vi "HFRR ADV v023 new software.vi"() -> ()   [LabVIEW 2025] (continued)
                  n3402 = property on="WS1.4" class="DigNum (strict)"("Caption.Text"=w4564) -> ()  [unwired: 2 in, 2 out]
                }
                frame 45 {
                  n3403 = property on="Save Results" class="Bool (strict)"("Boolean Text.Text"=w4566) -> ()  [unwired: 2 in, 2 out]
                }
                frame 46 {
                  n3404 = local write "S 47"(w4567) -> ()
                }
                frame 47 {
                  n3405 = local write "S 48"(w4568) -> ()
                }
                frame 48 {
                  n3406 = local write "S 49"(w4569) -> ()
                }
                frame 49 {
                  n3407 = local write "S 50"(w4570) -> ()
                }
                frame 50 {
                  n3408 = local write "S 51"(w4571) -> ()
                }
                frame 51 {
                  n3409 = local write "S 52"(w4572) -> ()
                }
                frame 52 {
                  n3410 = local write "S 53"(w4573) -> ()
                }
                frame 53 {
                  n3411 = local write "S 54"(w4574) -> ()
                }
                frame 54 {
                  n3412 = local write "S 55"(w4575) -> ()
                }
                frame 55 {
                  n3413 = local write "S 56"(w4576) -> ()
                }
                frame 56 {
                  n3414 = local write "S 57"(w4577) -> ()
                }
                frame 57 {
                  n3415 = local write "S 58"(w4578) -> ()
                }
                frame 58 {
                  n3416 = local write "S 59"(w4579) -> ()
                }
                frame 59 {
                  n3417 = local write "S 60"(w4580) -> ()
                }
                frame 60 {
                  n3418 = local write "S 62"(w4581) -> ()
                }
                frame 61 {
                  n3419 = local write "S 63"(w4582) -> ()
                }
                frame 62 {
                  n3420 = local write "S 64"(w4583) -> ()
                }
                frame 63 {
                  n3421 = local write "S 65"(w4584) -> ()
                }
                frame 64 {
                  n3422 = local write "S 66"(w4585) -> ()
                }
                frame 65 {
                  n3423 = local write "S 67"(w4586) -> ()
                }
                frame 66 {
                  n3424 = local write "S 68"(w4587) -> ()
                }
                frame 67 {
                  n3425 = local write "S 69"(w4588) -> ()
                }
                frame 68 {
                  n3426 = local write "S 70"(w4589) -> ()
                }
                frame 69 {
                  n3427 = local write "S 71"(w4590) -> ()
                }
                frame 70 {
                  n3428 = local write "S 72"(w4591) -> ()
                }
                frame 71 {
                  n3429 = local write "S 73"(w4592) -> ()
                }
                frame 72 {
                  n3430 = local write "S 74"(w4593) -> ()
                }
                frame 73 {
                  n3431 = local write "S 75"(w4594) -> ()
                }
                frame 74 {
                  n3432 = local write "S 76"(w4595) -> ()
                }
                frame 75 {
                  n3433 = local write "S 77"(w4596) -> ()
                }
                frame 76 {
                  n3434 = local write "S 78"(w4597) -> ()
                }
                frame 77 {
                  n3435 = local write "S 79"(w4598) -> ()
                }
                frame 79 {
                  n3436 = property on="Sample Temperature ( °C )" class="XYGraph (strict)"("Y Scale.Name Label.Text"=w4599) -> ()  [unwired: 2 in, 2 out]
                }
                frame 80 {
                  n3437 = local write "S 81"(w4600) -> ()
                  n3438 = property on="Humidity ( %RH )" class="XYGraph (strict)"("Y Scale.Name Label.Text"=w4600) -> ()  [unwired: 2 in, 2 out]
                }
                frame 78 {
                  n3439 = property on="Air Temperature  ( °C )" class="XYGraph (strict)"("X Scale.Name Label.Text"=w4601) -> ()  [unwired: 2 in, 2 out]
                  n3440 = property on="Humidity ( %RH )" class="XYGraph (strict)"("X Scale.Name Label.Text"=w4601) -> ()  [unwired: 2 in, 2 out]
                  n3441 = property on="Sample Temperature ( °C )" class="XYGraph (strict)"("X Scale.Name Label.Text"=w4601) -> ()  [unwired: 2 in, 2 out]
                  n3442 = property on="Coefficient Of Friction" class="XYGraph (strict)"("X Scale.Name Label.Text"=w4601) -> ()  [unwired: 2 in, 2 out]
                }
                frame 81 {
                  n3443 = property on="Air Temperature  ( °C )" class="XYGraph (strict)"("Y Scale.Name Label.Text"=w4602) -> ()  [unwired: 2 in, 2 out]
                }
                frame 82 {
                  n3444 = local write "S 84"(w4603) -> ()
                }
                frame 83 {
                  n3445 = local write "S 85"(w4604) -> ()
                }
                frame 84 {
                  n3446 = local write "S 86"(w4605) -> ()
                }
                frame 85 {
                  n3447 = local write "S 87"(w4606) -> ()
                }
                frame 86 {
                  n3448 = local write "S 88"(w4607) -> ()
                }
                frame 87 {
                }
                frame 88 {
                  n3449 = local write "S 90"(w4609) -> ()
                }
                frame 89 {
                  n3450 = local write "S 91"(w4610) -> ()
                }
                frame 90 {
                  n3451 = local write "S 92"(w4611) -> ()
                }
                frame 91 {
                  n3452 = local write "S 93"(w4612) -> ()
                }
                frame 92 {
                  n3453 = local write "S 94"(w4613) -> ()
                }
                frame 93 {
                  n3454 = local write "S 95"(w4614) -> ()
                }
                frame 94 {
                  n3455 = local write "S 96"(w4615) -> ()
                }
                frame 95 {
                  n3456 = local write "S 97"(w4616) -> ()
                }
                frame 96 {
                  n3457 = local write "S 98"(w4617) -> ()
                }
                frame 97 {
                  n3458 = local write "S 99"(w4618) -> ()
                }
                frame 98 {
                  n3459 = local write "S 100"(w4619) -> ()
                }
                frame 99 {
                  n3460 = local write "S 101"(w4620) -> ()
                }
                frame 100 {
                  n3461 = local write "S 102"(w4621) -> ()
                }
                frame 101 {
                  n3462 = local write "S 103"(w4622) -> ()
                }
                frame 102 {
                  n3463 = local write "S 104"(w4623) -> ()
                }
                frame 103 {
                  n3464 = local write "S 105"(w4624) -> ()
                }
                frame 104 {
                  n3465 = local write "S 106"(w4625) -> ()
                }
                frame 105 {
                }
                frame 106 {
                  n3466 = property on="OK Button 17" class="Bool (strict)"("Boolean Text.Text"=w4626) -> ()  [unwired: 2 in, 2 out]
                }
                frame 107 {
                  n3467 = property on="OK Button 16" class="Bool (strict)"("Boolean Text.Text"=w4627) -> ()  [unwired: 2 in, 2 out]
                }
                frame 108 {
                  n3468 = property on="TITTLE" class="Str"("Caption.Text"=w4628) -> ()  [unwired: 2 in, 2 out]
                }
                frame 109 {
                  "String 30" <- w4629
                }
                frame 110 {
                  n3469 = property on="Test Date" class="Str"("Caption.Text"=w4630) -> ()  [unwired: 2 in, 2 out]
                  "String 31" <- w4630
                }
                frame 111 {
                  n3470 = property on="Sample ID" class="Str"("Caption.Text"=w4631) -> ()  [unwired: 2 in, 2 out]
                  "String 32" <- w4631
                }
                frame 112 {
                  n3471 = property on="Tested by" class="Str"("Caption.Text"=w4632) -> ()  [unwired: 2 in, 2 out]
                  "String 33" <- w4632
                }
                frame 113 {
                  n3472 = property on="System Configured Printers 2" class="Arr (strict)"("Caption.Text"=w4633) -> ()  [unwired: 2 in, 2 out]
                }
                frame 114 {
                  n3473 = property on="Selected Printer" class="Str"("Caption.Text"=w4634) -> ()  [unwired: 2 in, 2 out]
                }
                frame 115 {
                  n3474 = property on="Select Printer 3" class="DigNum (strict)"("Caption.Text"=w4635) -> ()  [unwired: 2 in, 2 out]
                }
                frame 116 {
                  n3475 = property on="Print" class="Bool (strict)"("Boolean Text.Text"=w4636) -> ()  [unwired: 2 in, 2 out]
                }
                frame 117 {
                  "String 41" <- w4637
                }
                frame 118 {
                  n3476 = property on="tested by" class="Str"("Caption.Text"=w4638) -> ()  [unwired: 2 in, 2 out]
                }
                frame 119 {
                }
                frame 120 {
                  n3477 = property on="Export" class="Bool (strict)"("Boolean Text.Text"=w4639) -> ()  [unwired: 2 in, 2 out]
                }
                frame 121 {
                  n3478 = property on="TEMP INTERCEPT:" class="DigNum (strict)"("Caption.Text"=w4640) -> ()  [unwired: 2 in, 2 out]
                }
                frame 122 {
                  n3479 = property on="AIR TEMP INTERCEPT:" class="DigNum (strict)"("Caption.Text"=w4641) -> ()  [unwired: 2 in, 2 out]
                }
                frame 123 {
                  n3480 = property on="Select File Type" class="Enum (strict)"("Caption.Text"=w4642) -> ()  [unwired: 2 in, 2 out]
                }
                frame 124 {
                  n3481 = property on="s.NO" class="Str"("Caption.Text"=w4643) -> ()  [unwired: 2 in, 2 out]
                  "String 45" <- w4643
                }
                frame 125 {
                  n3482 = property on="trip1 8" class="Bool (strict)"("Boolean Text.Text"=w4644) -> ()  [unwired: 2 in, 2 out]
                }
                frame 126, Default {
                }
              }
            }
          }
          frame #1 {
            w4652 = TRUE ("Visible")
            n3483 = local read "S 91"() -> (w4669:string)
            n3484 = local read "S 90"() -> (w4668:string)
            n3485 = local read "S 88"() -> (w4667:string)
            n3486 = property on="File Path" class="Path"("Caption.Text"=w4668) -> ()  [unwired: 2 in, 2 out]
            n3487 = property on="SrvM CP" class="Bool (strict)"("Boolean Text.Text"=w4667) -> ()  [unwired: 2 in, 2 out]
            n3488 = local read "S 71"() -> (w4662:string)
            n3489 = local read "S 86"() -> (w4664:string)
            n3490 = local read "S 85"() -> (w4665:string)
            n3491 = local read "S 87"() -> (w4663:string)
            n3492 = local read "S 84"() -> (w4666:string)
            n3493 = local read "S 103"() -> (w4651:string)
            n3494 = local read "S 104"() -> (w4650:string)
            n3495 = property on="ENTER THE NEW PASSWORD" class="Str"("Caption.Text"=w4663) -> ()  [unwired: 2 in, 2 out]
            n3496 = property on="Password" class="Str"("Caption.Text"=w4665) -> ()  [unwired: 2 in, 2 out]
            n3497 = property on="ENTER CURRENT PASSWORD" class="Str"("Caption.Text"=w4664) -> ()  [unwired: 2 in, 2 out]
            n3498 = property on="EDIT" class="Bool (strict)"("Boolean Text.Text"=w4662) -> ()  [unwired: 2 in, 2 out]
            n3499 = property on="SAVE" class="Bool (strict)"("Boolean Text.Text"=w4666) -> ()  [unwired: 2 in, 2 out]
            n3500 = Build Array(w4651, w4650) -> (w4649:string[])
            n3501 = property on="Heater Button" class="Bool (strict)"("Strings [4]"=w4649) -> ()  [unwired: 2 in, 2 out]
            n3502 = property on="CH-HUMIDITY WET" class="DigNum (strict)"("Caption.Size to Text?"=w4652) -> ()  [unwired: 2 in, 2 out]
            n3503 = property on="CH-HUMIDITY DRY" class="DigNum (strict)"("Caption.Size to Text?"=w4652) -> ()  [unwired: 2 in, 2 out]
            n3504 = property on="CH-POWER -" class="DigNum (strict)"("Caption.Size to Text?"=w4652) -> ()  [unwired: 2 in, 2 out]
            n3505 = property on="CH-HEATER" class="DigNum (strict)"("Caption.Size to Text?"=w4652) -> ()  [unwired: 2 in, 2 out]
            n3506 = property on="CH-POWER +" class="DigNum (strict)"("Caption.Size to Text?"=w4652) -> ()  [unwired: 2 in, 2 out]
            n3507 = local read "S 92"() -> (w4661:string)
            n3508 = local read "S 93"() -> (w4660:string)
            n3509 = local read "S 105"() -> (w4647:string)
            n3510 = local read "S 106"() -> (w4646:string)
            n3511 = Build Array(w4661, w4660) -> ()  [unwired: 1 out]
            n3512 = Build Array(w4647, w4646) -> (w4648:string[])
            n3513 = local read "S 95"() -> (w4658:string)
            n3514 = local read "S 94"() -> (w4659:string)
            n3515 = local read "bs"() -> (w4674:string)
            n3516 = local read "as"() -> (w4675:string)
            n3517 = property on="Humidity" class="Bool (strict)"("Strings [4]"=w4648) -> ()  [unwired: 2 in, 2 out]
            n3518 = Concatenate Strings(w4674, "\r", w4675) -> ()  [unwired: 1 out]
            n3519 = property on="STROKE GAIN :" class="DigNum (strict)"("Caption.Text"=w4658) -> ()  [unwired: 2 in, 2 out]
            n3520 = property on="DISPLACEMENT :" class="DigNum (strict)"("Caption.Text"=w4659) -> ()  [unwired: 2 in, 2 out]
            n3521 = property on="Rh After" class="DigNum (strict)"("Caption.Size to Text?"=TRUE ("Caption.Size to Text")) -> ()  [unwired: 2 in, 2 out]
            n3522 = local read "S 48"() -> (w4698:string)
            n3523 = local read "S 50"() -> (w4696:string)
            n3524 = local read "S 51"() -> (w4695:string)
            n3525 = local read "S 49"() -> (w4697:string)
            n3526 = local read "S 52"() -> (w4694:string)
            n3527 = local read "as"() -> (w4679:string)
            n3528 = local read "bs"() -> (w4680:string)
            n3529 = local read "S 56"() -> (w4693:string)
            n3530 = local read "S 57"() -> (w4692:string)
            n3531 = local read "S 58"() -> (w4691:string)
            n3532 = local read "S 59"() -> (w4690:string)
            n3533 = property on="OPEN" class="Bool (strict)"("Boolean Text.Text"=w4694) -> ()  [unwired: 2 in, 2 out]
            n3534 = property on="OPEN 1" class="Bool (strict)"("Boolean Text.Text"=w4698) -> ()  [unwired: 2 in, 2 out]
            n3535 = property on="OPEN 2" class="Bool (strict)"("Boolean Text.Text"=w4697) -> ()  [unwired: 2 in, 2 out]
            n3536 = property on="OPEN 3" class="Bool (strict)"("Boolean Text.Text"=w4696) -> ()  [unwired: 2 in, 2 out]
            n3537 = property on="OPEN 4" class="Bool (strict)"("Boolean Text.Text"=w4695) -> ()  [unwired: 2 in, 2 out]
            n3538 = Concatenate Strings(w4680, "\r", w4679) -> ()  [unwired: 1 out]
            n3539 = local read "S 102"() -> (w4653:string)
            n3540 = property on="КОФ1" class="DigNum (strict)"("Caption.Text"=w4693) -> ()  [unwired: 2 in, 2 out]
            n3541 = local read "S 98"() -> (w4657:string)
            n3542 = local read "S 99"() -> (w4656:string)
            n3543 = local read "S 100"() -> (w4655:string)
            n3544 = local read "S 101"() -> (w4654:string)
            n3545 = property on="КОФ2" class="DigNum (strict)"("Caption.Text"=w4692) -> ()  [unwired: 2 in, 2 out]
            n3546 = property on="КОФ3" class="DigNum (strict)"("Caption.Text"=w4691) -> ()  [unwired: 2 in, 2 out]
            n3547 = property on="КОФ4" class="DigNum (strict)"("Caption.Text"=w4690) -> ()  [unwired: 2 in, 2 out]
            n3548 = local read "bs"() -> (w4678:string)
            n3549 = local read "as"() -> (w4677:string)
            n3550 = property on="CH-POWER +" class="DigNum (strict)"("Caption.Text"=w4657) -> ()  [unwired: 2 in, 2 out]
            n3551 = property on="CH-POWER -" class="DigNum (strict)"("Caption.Text"=w4656) -> ()  [unwired: 2 in, 2 out]
            n3552 = property on="CH-HEATER" class="DigNum (strict)"("Caption.Text"=w4655) -> ()  [unwired: 2 in, 2 out]
            n3553 = property on="CH-HUMIDITY DRY" class="DigNum (strict)"("Caption.Text"=w4654) -> ()  [unwired: 2 in, 2 out]
            n3554 = property on="CH-HUMIDITY WET" class="DigNum (strict)"("Caption.Text"=w4653) -> ()  [unwired: 2 in, 2 out]
            n3555 = local read "S 60"() -> (w4689:string)
            n3556 = local read "S 54"() -> (w4699:string)
            n3557 = Concatenate Strings(w4678, "\r", w4677) -> ()  [unwired: 1 out]
            n3558 = Concatenate Strings(w4699, w4689) -> ()  [unwired: 1 out]
            n3559 = local read "S 77"() -> (→"String 43":string)
            n3560 = local read "S 76"() -> (w4672:string)
            n3561 = local read "S 78"() -> (w4671:string)
            n3562 = local read "S 71"() -> (w4683:string)
            n3563 = local read "S 66"() -> (w4688:string)
            n3564 = local read "S 67"() -> (w4687:string)
            n3565 = local read "S 68"() -> (w4686:string)
            n3566 = local read "S 69"() -> (w4685:string)
            n3567 = local read "S 70"() -> (w4684:string)
            n3568 = property on="AIR TEMP" class="DigNum (strict)"("Caption.Text"=w4671) -> ()  [unwired: 2 in, 2 out]
            n3569 = property on="Set Strk" class="DigNum (strict)"("Caption.Text"=w4672) -> ()  [unwired: 2 in, 2 out]
            n3570 = property on="FRIC. FORCE :" class="DigNum (strict)"("Caption.Text"=w4688) -> ()  [unwired: 2 in, 2 out]
            n3571 = property on="TEMPERATURE :" class="DigNum (strict)"("Caption.Text"=w4687) -> ()  [unwired: 2 in, 2 out]
            n3572 = property on="SPEED OUT:" class="DigNum (strict)"("Caption.Text"=w4686) -> ()  [unwired: 2 in, 2 out]
            n3573 = property on="AIR TEMPERATURE :" class="DigNum (strict)"("Caption.Text"=w4685) -> ()  [unwired: 2 in, 2 out]
            n3574 = property on="HUMIDITY:" class="DigNum (strict)"("Caption.Text"=w4684) -> ()  [unwired: 2 in, 2 out]
            n3575 = property on="EDIT" class="Bool (strict)"("Boolean Text.Text"=w4683) -> ()  [unwired: 2 in, 2 out]
            n3576 = local read "S 79"() -> (w4670:string)
          }
          frame #2 {
          }
        }
        n3577 = local write "Lan flag"(10.0 ("Lan flag")) -> ()
      }
      frame Enabled {
      }
    }
    n3578 = Wait (ms)(milliseconds to wait=u32 2000) -> ()  [unwired: 1 out]
    n3579 = local read "Quit"() -> (w4473:bool)
  }
  n3580 = while {
    shift-right: [w4705] -> _
    shift-left: _ -> [w4706]
    shift-right: [w4703] -> _
    shift-left: T18 {"Read Heave and Surge"="", "Bytes at Heave Port"=0.0, "Heave and Surge COM Port:"="COM9", "Com Port 2"="COM7", "Residual Due"="", "Heave COM Status 2"=TRUE, "Heave COM Status"=TRUE, "Port 2"=TRUE, "Sway PPR"=6400.0, "Surge PPR"=6400.0, "Heave PPR"=6400.0, "Sway Pitch"=2.0, "Surge Pitch"=3.0, "Heave Pitch"=4.0, "Sway Pulses/mm"=320.0, "Surge Pulses/mm"=1600.0, "Heave Pulses/mm"=1600.0, "inner loop"=0.0, "Read Heave and Surge 2"="", "String 36"="", "Write S"=FALSE, "WriteCC1"=[""], "Heave COM Loop"=0, "LastCom"="", "EXIT"=FALSE, "Error Heave"={"status"=TRUE, "code"=-1073807343, "source"=""}} -> [w4702]
    shift-right: [w4700] -> _
    shift-left: enum16{"init", "MAIN", "Panel Close"}."init" -> [w4701]
    stop <- w4704 stop-if-true
    n3581 = case shown="\"MAIN\"" w4701 {
      tunnel: w4706 -> [w4720 w4736 w4796 w4798]
      tunnel: [w4715 w4744 w4796 w4798] -> w4705
      tunnel: [_ _ TRUE _] -> w4704
      tunnel: [w4711 w4742 w4794 w4797] -> w4703
      tunnel: w4702 -> [w4717 w4735 w4794 w4797]
      tunnel: [enum16{"init", "MAIN", "Panel Close"}."MAIN" w4730 _ _] -> w4700
      frame "init" {
        n3582 = local read "Com Port 1"() -> (w4707:refnum<visa-resource-name>)
        n3583 = Bundle By Name(cluster=w4717, "Heave and Surge COM Port:"=w4707) -> (w4716:T18)
        n3584 = call "Instrument fgv uno.vi"("Enum"=T31."INIT", "error in (no error) 2"=w4720, "INPUT"=w4716) -> ("error"=w4718:errorcluster, "output"=w4714:T18)  [unwired: 6 in, 1 out]
        n3585 = case shown="Error" w4718 {
          selector: w4718 -> [w4722 _]
          tunnel: [w4722 w4726] -> w4715
          tunnel: w4714 -> [w4721 w4724]
          tunnel: [w4721 w4723] -> w4712
          frame No Error {
          }
          frame Error {
            n3586 = call "Instrument fgv uno.vi"("Enum"=T31."ERROR INIT", "INPUT"=w4724) -> ("error"=w4727:errorcluster, "output"=w4723:T18)  [unwired: 7 in, 1 out]
            n3587 = call <vilib>:"Clear Errors.vi"("error in (no error)"=w4727) -> ("error out"=w4726:errorcluster)  [unwired: 5 in, 1 out]
          }
        }
        n3588 = local read "LastCom 2"() -> (w4710:string)
        n3589 = Unbundle By Name(w4712) -> ("Heave COM Status 2"=→"COM Status 2" →"Instrument Status 2":bool, "Error Heave"=→"Error  2":errorcluster)  [unwired: 1 out]
        n3590 = Bundle By Name(cluster=w4712, "LastCom"=w4710) -> (w4711:T18)
      }
      frame "MAIN" {
        n3591 = Unbundle By Name(w4735) -> ("Com Port 2"=w4746:refnum<visa-resource-name>)
        n3592 = local read "Com Port 1"() -> (w4729:refnum<visa-resource-name>)
        n3593 = local write "Com Port 5"(w4746) -> ()
        n3594 = Bundle By Name(cluster=w4735, "Heave and Surge COM Port:"=w4729) -> (w4734:T18)
        n3595 = Equal?(x=w4746, y=w4729) -> (x = y?=w4745:bool)
        n3596 = case shown="True" w4745 {
          tunnel: [w4750 w4767] -> w4744
          tunnel: w4736 -> [w4751 w4773]
          tunnel: w4734 -> [w4749 w4771]
          tunnel: [w4748 w4766] -> w4742
          frame False {
            n3597 = call <vilib>:"Clear Errors.vi"("error in (no error)"=w4751) -> ("error out"=w4747:errorcluster)  [unwired: 5 in, 1 out]
            n3598 = call "Instrument fgv uno.vi"("Enum"=T31."ERROR INIT", "error in (no error) 2"=w4747, "INPUT"=w4749) -> ("error"=w4753:errorcluster, "output"=w4748:T18)  [unwired: 6 in, 1 out]
            n3599 = call <vilib>:"Clear Errors.vi"("error in (no error)"=w4753) -> ("error out"=w4750:errorcluster)  [unwired: 5 in, 1 out]
          }
          frame True {
            n3600 = call "Instrument fgv uno.vi"("Enum"=T31."READ", "error in (no error) 2"=w4773, "INPUT"=w4771) -> ("error"=w4772:errorcluster, "output"=w4763:T18)  [unwired: 6 in, 1 out]
            n3601 = Bundle By Name(cluster=w4763, "String 36"="String 15") -> (w4762:T18)
            n3602 = case shown="True" "Write S 2" {
              selector: "Write S 2" -> [_ w4793]
              tunnel: w4772 -> [w4786 w4792]
              tunnel: [w4786 w4791] -> w4759
              tunnel: w4762 -> [w4785 w4788]
              tunnel: [w4785 w4787] -> w4758
              frame False {
              }
              frame True {
                n3603 = Not(x=w4793) -> (.not. x?=w4789:bool)
                n3604 = local write "Write S 2"(w4789) -> ()
                n3605 = call "Instrument fgv uno.vi"("Enum"=T31."MANUAL WRITE", "error in (no error) 2"=w4792, "INPUT"=w4788) -> ("error"=w4791:errorcluster, "output"=w4787:T18)  [unwired: 6 in, 1 out]
              }
            }
            n3606 = Array Size(array="WriteHumidity") -> (size(s)=w4756:i32)
            n3607 = Greater Than 0?(x=w4756) -> (x > 0?=w4755:bool)
            n3608 = call "Instrument fgv uno.vi"("Enum"=T31."WRITE", "error in (no error) 2"=w4759, "WriteCC1"="WriteHumidity", "INPUT"=w4758) -> ("error"=w4769:errorcluster, "WriteCC1 2"=w4757:string[], "output"=w4768:T18)  [unwired: 5 in]
            n3609 = case shown="True" w4755 {
              tunnel: w4757 -> [_ w4775]
              frame False {
              }
              frame True {
                n3610 = local write "WriteHumidity 2"(w4775) -> ()
              }
            }
            n3611 = case shown="No Error" w4769 {
              selector: w4769 -> [w4776 w4779]
              tunnel: w4768 -> [w4777 w4784]
              tunnel: [w4777 w4783] -> w4766
              tunnel: [w4776 w4781] -> w4767
              frame No Error {
              }
              frame Error {
                n3612 = call <vilib>:"Clear Errors.vi"("error in (no error)"=w4779) -> ("error out"=w4778:errorcluster)  [unwired: 5 in, 1 out]
                n3613 = call "Instrument fgv uno.vi"("Enum"=T31."ERROR INIT", "error in (no error) 2"=w4778, "INPUT"=w4784) -> ("error"=w4782:errorcluster, "output"=w4783:T18)  [unwired: 6 in, 1 out]
                n3614 = call <vilib>:"Clear Errors.vi"("error in (no error)"=w4782) -> ("error out"=w4781:errorcluster)  [unwired: 5 in, 1 out]
              }
            }
            n3615 = Unbundle By Name(w4766) -> ("LastCom"=→"LastCom 2":string, "Read Heave and Surge"=→"Read Uno":string)
          }
        }
        n3616 = Unbundle By Name(w4742) -> ("Heave COM Status 2"=w4743:bool, "Heave COM Status"=w4728:bool, "Error Heave"=w4740:errorcluster, "Bytes at Heave Port"=→"Bytes at Humidity Port  2":dbl)
        n3617 = Unbundle By Name(w4740) -> ("status"=→"Humidity Port 2":bool)
        n3618 = Not(x=w4728) -> (.not. x?=w4737:bool)
        n3619 = local write "Error  2"(w4740) -> ()
        n3620 = Not(x=w4743) -> (.not. x?=w4738:bool)
        n3621 = local write "Instrument Status 2"(w4737) -> ()
        n3622 = local write "COM Status 2"(w4738) -> ()
        n3623 = local write "Port 1a"(w4728) -> ()
        n3624 = local read "Quit"() -> (w4731:bool)
        n3625 = Select(t=enum16{"init", "MAIN", "Panel Close"}."Panel Close", s=w4731, f=enum16{"init", "MAIN", "Panel Close"}."MAIN") -> (s? t:f=w4730:enum16{"init", "MAIN", "Panel Close"})
      }
      frame "Panel Close" {
      }
      frame Default {
      }
    }
  }
  n3626 = disable-structure shown="Disabled" {
    frame Disabled {
      n3627 = while {
        tunnel: [w4800] -> _
        i -> [w4800]
        stop <- w4799 continue-if-true
        n3628 = Wait (ms)(milliseconds to wait=u32 50) -> ()  [unwired: 1 out]
        n3629 = stacked-sequence {
          frame #0 {
            # "Controls Text color"
            # "Controls BG color"
            n3630 = property on="FILE" class="Str"("Text.Text Colors:Text Color"="SC  Text") -> ()  [unwired: 2 in, 2 out]
            n3631 = property on="Fuel Discription :" class="Str"("Text.Text Colors:Text Color"="SC  Text") -> ()  [unwired: 2 in, 2 out]
            n3632 = property on="tested by" class="Str"("Text.Text Colors:Text Color"="SC  Text") -> ()  [unwired: 2 in, 2 out]
            n3633 = property on="Remarks :" class="Str"("Text.Text Colors:Text Color"="SC  Text") -> ()  [unwired: 2 in, 2 out]
            n3634 = property class="DigNum (strict)"("Numeric Text.Text Colors:BG Color"="NC BG") -> ()  [unwired: 2 in, 2 out]
            n3635 = property class="DigNum (strict)"("Numeric Text.Text Colors:BG Color"="NC BG") -> ()  [unwired: 2 in, 2 out]
            n3636 = property class="DigNum (strict)"("Numeric Text.Text Colors:BG Color"="NC BG") -> ()  [unwired: 2 in, 2 out]
            n3637 = property class="DigNum (strict)"("Numeric Text.Text Colors:BG Color"="NC BG") -> ()  [unwired: 2 in, 2 out]
            n3638 = property class="DigNum (strict)"("Numeric Text.Text Colors:BG Color"="NC BG") -> ()  [unwired: 2 in, 2 out]
            n3639 = property class="DigNum (strict)"("Numeric Text.Text Colors:BG Color"="NC BG") -> ()  [unwired: 2 in, 2 out]
            n3640 = property class="DigNum (strict)"("Numeric Text.Text Colors:BG Color"="NC BG") -> ()  [unwired: 2 in, 2 out]
            n3641 = property class="DigNum (strict)"("Numeric Text.Text Colors:BG Color"="NC BG") -> ()  [unwired: 2 in, 2 out]
            n3642 = property class="DigNum (strict)"("Numeric Text.Text Colors:BG Color"="NC BG") -> ()  [unwired: 2 in, 2 out]
            n3643 = property class="DigNum (strict)"("Numeric Text.Text Colors:BG Color"="NC BG") -> ()  [unwired: 2 in, 2 out]
            n3644 = property class="DigNum (strict)"("Numeric Text.Text Colors:BG Color"="NC BG") -> ()  [unwired: 2 in, 2 out]
            n3645 = property class="DigNum (strict)"("Numeric Text.Text Colors:BG Color"="NC BG") -> ()  [unwired: 2 in, 2 out]
            n3646 = property on="FILE" class="Str"("Text.Text Colors:BG Color"="SC BG 3") -> ()  [unwired: 2 in, 2 out]
            n3647 = property on="Fuel Discription :" class="Str"("Text.Text Colors:BG Color"="SC BG 3") -> ()  [unwired: 2 in, 2 out]
            n3648 = property on="tested by" class="Str"("Text.Text Colors:BG Color"="SC BG 3") -> ()  [unwired: 2 in, 2 out]
            n3649 = property on="Remarks :" class="Str"("Text.Text Colors:BG Color"="SC BG 3") -> ()  [unwired: 2 in, 2 out]
            n3650 = property class="DigNum (strict)"("Numeric Text.Text Colors:Text Color"="NC Text") -> ()  [unwired: 2 in, 2 out]
            n3651 = property class="DigNum (strict)"("Numeric Text.Text Colors:Text Color"="NC Text") -> ()  [unwired: 2 in, 2 out]
            n3652 = property class="DigNum (strict)"("Numeric Text.Text Colors:Text Color"="NC Text") -> ()  [unwired: 2 in, 2 out]
            n3653 = property class="DigNum (strict)"("Numeric Text.Text Colors:Text Color"="NC Text") -> ()  [unwired: 2 in, 2 out]
            n3654 = property class="DigNum (strict)"("Numeric Text.Text Colors:Text Color"="NC Text") -> ()  [unwired: 2 in, 2 out]
            n3655 = property class="DigNum (strict)"("Numeric Text.Text Colors:Text Color"="NC Text") -> ()  [unwired: 2 in, 2 out]
            n3656 = property class="DigNum (strict)"("Numeric Text.Text Colors:Text Color"="NC Text") -> ()  [unwired: 2 in, 2 out]
            n3657 = property class="DigNum (strict)"("Numeric Text.Text Colors:Text Color"="NC Text") -> ()  [unwired: 2 in, 2 out]
            n3658 = property class="DigNum (strict)"("Numeric Text.Text Colors:Text Color"="NC Text") -> ()  [unwired: 2 in, 2 out]
            n3659 = property class="DigNum (strict)"("Numeric Text.Text Colors:Text Color"="NC Text") -> ()  [unwired: 2 in, 2 out]
            n3660 = property class="DigNum (strict)"("Numeric Text.Text Colors:Text Color"="NC Text") -> ()  [unwired: 2 in, 2 out]
            n3661 = property class="DigNum (strict)"("Numeric Text.Text Colors:Text Color"="NC Text") -> ()  [unwired: 2 in, 2 out]
            n3662 = property class="DigNum (strict)"("Numeric Text.Text Colors:Text Color"="NI Text  2") -> ()  [unwired: 2 in, 2 out]
            n3663 = property class="DigNum (strict)"("Numeric Text.Text Colors:Text Color"="NI Text  2") -> ()  [unwired: 2 in, 2 out]
            n3664 = property class="DigNum (strict)"("Numeric Text.Text Colors:Text Color"="NI Text  2") -> ()  [unwired: 2 in, 2 out]
            n3665 = property class="DigNum (strict)"("Numeric Text.Text Colors:Text Color"="NI Text  2") -> ()  [unwired: 2 in, 2 out]
            n3666 = property class="DigNum (strict)"("Numeric Text.Text Colors:Text Color"="NI Text  2") -> ()  [unwired: 2 in, 2 out]
            n3667 = property class="DigNum (strict)"("Numeric Text.Text Colors:Text Color"="NI Text  2") -> ()  [unwired: 2 in, 2 out]
            n3668 = property class="DigNum (strict)"("Numeric Text.Text Colors:Text Color"="NI Text  2") -> ()  [unwired: 2 in, 2 out]
            n3669 = property class="DigNum (strict)"("Numeric Text.Text Colors:Text Color"="NI Text  2") -> ()  [unwired: 2 in, 2 out]
            n3670 = property class="DigNum (strict)"("Numeric Text.Text Colors:Text Color"="NI Text  2") -> ()  [unwired: 2 in, 2 out]
            n3671 = property class="DigNum (strict)"("Numeric Text.Text Colors:Text Color"="NI Text  2") -> ()  [unwired: 2 in, 2 out]
            n3672 = property class="DigNum (strict)"("Numeric Text.Text Colors:Text Color"="NI Text  2") -> ()  [unwired: 2 in, 2 out]
            n3673 = property class="DigNum (strict)"("Numeric Text.Text Colors:Text Color"="NI Text  2") -> ()  [unwired: 2 in, 2 out]
            n3674 = property class="DigNum (strict)"("Numeric Text.Text Colors:Text Color"="NI Text  2") -> ()  [unwired: 2 in, 2 out]
            n3675 = property class="DigNum (strict)"("Numeric Text.Text Colors:Text Color"="NI Text  2") -> ()  [unwired: 2 in, 2 out]
            n3676 = property class="DigNum (strict)"("Numeric Text.Text Colors:Text Color"="NI Text  2") -> ()  [unwired: 2 in, 2 out]
            n3677 = property on="Coefficient Of Friction" class="XYGraph (strict)"("Plot Area:Colors:FG Color"="GFG  2", "Plot Area:Colors:BG Color"="GBG   2") -> ()  [unwired: 2 in, 2 out]
            n3678 = property on="Humidity ( %RH )" class="XYGraph (strict)"("Plot Area:Colors:FG Color"="GFG  2", "Plot Area:Colors:BG Color"="GBG   2") -> ()  [unwired: 2 in, 2 out]
            n3679 = property on="Air Temperature  ( °C )" class="XYGraph (strict)"("Plot Area:Colors:FG Color"="GFG  2", "Plot Area:Colors:BG Color"="GBG   2") -> ()  [unwired: 2 in, 2 out]
            n3680 = property on="Sample Temperature ( °C )" class="XYGraph (strict)"("Plot Area:Colors:FG Color"="GFG  2", "Plot Area:Colors:BG Color"="GBG   2") -> ()  [unwired: 2 in, 2 out]
            n3681 = property class="DigNum (strict)"("Numeric Text.Text Colors:BG Color"="NI BG 2") -> ()  [unwired: 2 in, 2 out]
            n3682 = property class="DigNum (strict)"("Numeric Text.Text Colors:BG Color"="NI BG 2") -> ()  [unwired: 2 in, 2 out]
            n3683 = property class="DigNum (strict)"("Numeric Text.Text Colors:BG Color"="NI BG 2") -> ()  [unwired: 2 in, 2 out]
            n3684 = property class="DigNum (strict)"("Numeric Text.Text Colors:BG Color"="NI BG 2") -> ()  [unwired: 2 in, 2 out]
            n3685 = property class="DigNum (strict)"("Numeric Text.Text Colors:BG Color"="NI BG 2") -> ()  [unwired: 2 in, 2 out]
            n3686 = property class="DigNum (strict)"("Numeric Text.Text Colors:BG Color"="NI BG 2") -> ()  [unwired: 2 in, 2 out]
            n3687 = property class="DigNum (strict)"("Numeric Text.Text Colors:BG Color"="NI BG 2") -> ()  [unwired: 2 in, 2 out]
            n3688 = property class="DigNum (strict)"("Numeric Text.Text Colors:BG Color"="NI BG 2") -> ()  [unwired: 2 in, 2 out]
            n3689 = property class="DigNum (strict)"("Numeric Text.Text Colors:BG Color"="NI BG 2") -> ()  [unwired: 2 in, 2 out]
            n3690 = property class="DigNum (strict)"("Numeric Text.Text Colors:BG Color"="NI BG 2") -> ()  [unwired: 2 in, 2 out]
            n3691 = property class="DigNum (strict)"("Numeric Text.Text Colors:BG Color"="NI BG 2") -> ()  [unwired: 2 in, 2 out]
            n3692 = property class="DigNum (strict)"("Numeric Text.Text Colors:BG Color"="NI BG 2") -> ()  [unwired: 2 in, 2 out]
            n3693 = property class="DigNum (strict)"("Numeric Text.Text Colors:BG Color"="NI BG 2") -> ()  [unwired: 2 in, 2 out]
            n3694 = property class="DigNum (strict)"("Numeric Text.Text Colors:BG Color"="NI BG 2") -> ()  [unwired: 2 in, 2 out]
            n3695 = property class="DigNum (strict)"("Numeric Text.Text Colors:BG Color"="NI BG 2") -> ()  [unwired: 2 in, 2 out]
            n3696 = property class="Bool"("Colors [4]"="Boolean BC T & BG") -> ()  [unwired: 2 in, 2 out]
            n3697 = property on="Save & Continue" class="Bool (strict)"("Colors [4]"="Boolean BC T & BG") -> ()  [unwired: 2 in, 2 out]
            n3698 = property on="Heater Button" class="Bool (strict)"("Colors [4]"="Boolean BC T & BG") -> ()  [unwired: 2 in, 2 out]
            n3699 = property class="Bool"("Colors [4]"="Boolean BC T & BG") -> ()  [unwired: 2 in, 2 out]
            n3700 = property on="Humidity" class="Bool (strict)"("Colors [4]"="Boolean BC T & BG") -> ()  [unwired: 2 in, 2 out]
            n3701 = property class="Bool (strict)"("Colors [4]"="Boolean BC T & BG") -> ()  [unwired: 2 in, 2 out]
            n3702 = property on="RUN" class="Bool (strict)"("Colors [4]"="Boolean BC T & BG") -> ()  [unwired: 2 in, 2 out]
            n3703 = property on="trip1 8" class="Bool (strict)"("Colors [4]"="Boolean BC T & BG") -> ()  [unwired: 2 in, 2 out]
            n3704 = property class="Bool"("Colors [4]"="Boolean BC T & BG") -> ()  [unwired: 2 in, 2 out]
            n3705 = property class="Bool (strict)"("Colors [4]"="Boolean BC T & BG") -> ()  [unwired: 2 in, 2 out]
            n3706 = property on="OPEN 1" class="Bool (strict)"("Colors [4]"="Boolean BC T & BG 2") -> ()  [unwired: 2 in, 2 out]
            n3707 = property on="OPEN 2" class="Bool (strict)"("Colors [4]"="Boolean BC T & BG 2") -> ()  [unwired: 2 in, 2 out]
            n3708 = property on="OPEN 3" class="Bool (strict)"("Colors [4]"="Boolean BC T & BG 2") -> ()  [unwired: 2 in, 2 out]
            n3709 = property on="OPEN 4" class="Bool (strict)"("Colors [4]"="Boolean BC T & BG 2") -> ()  [unwired: 2 in, 2 out]
            n3710 = property on="OPEN" class="Bool (strict)"("Colors [4]"="Boolean BC T & BG 2") -> ()  [unwired: 2 in, 2 out]
            n3711 = property on="rstv2" class="Bool"("Colors [4]"="Boolean BC T & BG 2") -> ()  [unwired: 2 in, 2 out]
            n3712 = property on="RST CP" class="Bool"("Colors [4]"="Boolean BC T & BG 2") -> ()  [unwired: 2 in, 2 out]
            n3713 = property on="RSTV1 3" class="Bool"("Colors [4]"="Boolean BC T & BG 2") -> ()  [unwired: 2 in, 2 out]
            n3714 = property on="RSTV1 2" class="Bool"("Colors [4]"="Boolean BC T & BG 2") -> ()  [unwired: 2 in, 2 out]
          }
          frame #1 {
          }
        }
        n3715 = local read "Quit"() -> (w4799:bool)
      }
    }
    frame Enabled {
    }
  }
  n3716 = while {
    shift-right: [w4817] -> _
    shift-left: _ -> [w4818]
    shift-right: [w4815] -> _
    shift-left: T18 {"Read Heave and Surge"="", "Bytes at Heave Port"=0.0, "Heave and Surge COM Port:"="COM9", "Com Port 2"="COM7", "Residual Due"="", "Heave COM Status 2"=TRUE, "Heave COM Status"=TRUE, "Port 2"=TRUE, "Sway PPR"=6400.0, "Surge PPR"=6400.0, "Heave PPR"=6400.0, "Sway Pitch"=2.0, "Surge Pitch"=3.0, "Heave Pitch"=4.0, "Sway Pulses/mm"=320.0, "Surge Pulses/mm"=1600.0, "Heave Pulses/mm"=1600.0, "inner loop"=0.0, "Read Heave and Surge 2"="", "String 36"="", "Write S"=FALSE, "WriteCC1"=[""], "Heave COM Loop"=0, "LastCom"="", "EXIT"=FALSE, "Error Heave"={"status"=TRUE, "code"=-1073807343, "source"=""}} -> [w4814]
    shift-right: [w4812] -> _
    shift-left: enum16{"init", "MAIN", "Panel Close"}."init" -> [w4813]
    stop <- w4816 stop-if-true
    n3717 = case shown="\"MAIN\"" w4813 {
      tunnel: w4818 -> [w4832 w4847 w4908 w4910]
      tunnel: [w4826 w4856 w4908 w4910] -> w4817
      tunnel: [_ _ TRUE _] -> w4816
      tunnel: [w4822 w4853 w4906 w4909] -> w4815
      tunnel: w4814 -> [w4829 w4846 w4906 w4909]
      tunnel: [enum16{"init", "MAIN", "Panel Close"}."MAIN" w4840 _ _] -> w4812
      frame "init" {
        n3718 = Bundle By Name(cluster=w4829, "Heave and Surge COM Port:"="C3 :") -> (w4828:T18)
        n3719 = call "Instrument fgv.vi"("Enum"=T31."INIT", "error in (no error) 2"=w4832, "INPUT"=w4828) -> ("error"=w4830:errorcluster, "output"=w4825:T18)  [unwired: 6 in, 1 out]
        n3720 = case shown="Error" w4830 {
          selector: w4830 -> [w4834 _]
          tunnel: [w4834 w4838] -> w4826
          tunnel: w4825 -> [w4833 w4836]
          tunnel: [w4833 w4835] -> w4823
          frame No Error {
          }
          frame Error {
            n3721 = call "Instrument fgv.vi"("Enum"=T31."ERROR INIT", "INPUT"=w4836) -> ("error"=w4839:errorcluster, "output"=w4835:T18)  [unwired: 7 in, 1 out]
            n3722 = call <vilib>:"Clear Errors.vi"("error in (no error)"=w4839) -> ("error out"=w4838:errorcluster)  [unwired: 5 in, 1 out]
          }
        }
        n3723 = local read "LastCom"() -> (w4821:string)
        n3724 = Unbundle By Name(w4823) -> ("Heave COM Status 2"=→"COM Status" →"Instrument Status":bool, "Error Heave"=→"Error":errorcluster)  [unwired: 1 out]
        n3725 = Bundle By Name(cluster=w4823, "LastCom"=w4821) -> (w4822:T18)
      }
      frame "MAIN" {
        n3726 = Unbundle By Name(w4846) -> ("Com Port 2"=w4858:refnum<visa-resource-name>)
        n3727 = local write "Com Port 4"(w4858) -> ()
        n3728 = local read "C3 :"() -> (w4844:refnum<visa-resource-name>)
        n3729 = Bundle By Name(cluster=w4846, "Heave and Surge COM Port:"=w4844) -> (w4845:T18)
        n3730 = Equal?(x=w4858, y=w4844) -> (x = y?=w4857:bool)
        n3731 = case shown="True" w4857 {
          tunnel: [w4862 w4879] -> w4856
          tunnel: w4847 -> [w4863 w4885]
          tunnel: w4845 -> [w4861 w4883]
          tunnel: [w4860 w4878] -> w4853
          frame False {
            n3732 = call <vilib>:"Clear Errors.vi"("error in (no error)"=w4863) -> ("error out"=w4859:errorcluster)  [unwired: 5 in, 1 out]
            n3733 = call "Instrument fgv.vi"("Enum"=T31."ERROR INIT", "error in (no error) 2"=w4859, "INPUT"=w4861) -> ("error"=w4865:errorcluster, "output"=w4860:T18)  [unwired: 6 in, 1 out]
            n3734 = call <vilib>:"Clear Errors.vi"("error in (no error)"=w4865) -> ("error out"=w4862:errorcluster)  [unwired: 5 in, 1 out]
          }
          frame True {
            n3735 = call "Instrument fgv.vi"("Enum"=T31."READ", "error in (no error) 2"=w4885, "INPUT"=w4883) -> ("error"=w4884:errorcluster, "output"=w4875:T18)  [unwired: 6 in, 1 out]
            n3736 = Bundle By Name(cluster=w4875, "String 36"="String 11") -> (w4874:T18)
            n3737 = case shown="True" "Write S" {
              selector: "Write S" -> [_ w4905]
              tunnel: w4884 -> [w4898 w4904]
              tunnel: [w4898 w4903] -> w4871
              tunnel: w4874 -> [w4897 w4900]
              tunnel: [w4897 w4899] -> w4870
              frame False {
              }
              frame True {
                n3738 = Not(x=w4905) -> (.not. x?=w4901:bool)
                n3739 = local write "Write S"(w4901) -> ()
                n3740 = call "Instrument fgv.vi"("Enum"=T31."MANUAL WRITE", "error in (no error) 2"=w4904, "INPUT"=w4900) -> ("error"=w4903:errorcluster, "output"=w4899:T18)  [unwired: 6 in, 1 out]
              }
            }
            n3741 = Array Size(array="WriteHumidity 2") -> (size(s)=w4868:i32)
            n3742 = Greater Than 0?(x=w4868) -> (x > 0?=w4867:bool)
            n3743 = call "Instrument fgv.vi"("Enum"=T31."WRITE", "error in (no error) 2"=w4871, "WriteCC1"="WriteHumidity 2", "INPUT"=w4870) -> ("error"=w4881:errorcluster, "WriteCC1 2"=w4869:string[], "output"=w4880:T18)  [unwired: 5 in]
            n3744 = case shown="True" w4867 {
              tunnel: w4869 -> [_ w4887]
              frame False {
              }
              frame True {
                n3745 = local write "WriteHumidity 2"(w4887) -> ()
              }
            }
            n3746 = case shown="Error" w4881 {
              selector: w4881 -> [w4888 w4891]
              tunnel: w4880 -> [w4889 w4896]
              tunnel: [w4889 w4895] -> w4878
              tunnel: [w4888 w4893] -> w4879
              frame No Error {
              }
              frame Error {
                n3747 = call <vilib>:"Clear Errors.vi"("error in (no error)"=w4891) -> ("error out"=w4890:errorcluster)  [unwired: 5 in, 1 out]
                n3748 = call "Instrument fgv.vi"("Enum"=T31."ERROR INIT", "error in (no error) 2"=w4890, "INPUT"=w4896) -> ("error"=w4894:errorcluster, "output"=w4895:T18)  [unwired: 6 in, 1 out]
                n3749 = call <vilib>:"Clear Errors.vi"("error in (no error)"=w4894) -> ("error out"=w4893:errorcluster)  [unwired: 5 in, 1 out]
              }
            }
            n3750 = Unbundle By Name(w4878) -> ("LastCom"=→"LastCom":string, "Read Heave and Surge"=→"Read Humidity":string)
          }
        }
        n3751 = Unbundle By Name(w4853) -> ("Heave COM Status 2"=w4855:bool, "Heave COM Status"=w4854:bool, "Error Heave"=w4851:errorcluster, "Bytes at Heave Port"=→"Bytes at Humidity Port":dbl)
        n3752 = Unbundle By Name(w4851) -> ("status"=→"Humidity Port":bool)
        n3753 = Not(x=w4854) -> (.not. x?=w4848:bool)
        n3754 = local write "Error"(w4851) -> ()
        n3755 = Not(x=w4855) -> (.not. x?=w4849:bool)
        n3756 = local write "Instrument Status"(w4848) -> ()
        n3757 = local write "COM Status"(w4849) -> ()
        n3758 = local read "Quit"() -> (w4841:bool)
        n3759 = Select(t=enum16{"init", "MAIN", "Panel Close"}."Panel Close", s=w4841, f=enum16{"init", "MAIN", "Panel Close"}."MAIN") -> (s? t:f=w4840:enum16{"init", "MAIN", "Panel Close"})
      }
      frame "Panel Close" {
      }
      frame Default {
      }
    }
  }
  n3760 = while {
    stop <- w4936 stop-if-true
    n3761 = local read "Read Uno"() -> (w4911:string)
    n3762 = call <vilib>:"High Resolution Polling Wait.vi"("seconds to wait"=0.05) -> ()  [unwired: 10 in, 1 out]
    n3763 = Spreadsheet String To Array(delimiter (Tab)=",", format string="", spreadsheet string=w4911, array type (2D Dbl)=string[] []) -> (array=w4931:string[])
    n3764 = for {
      tunnel: w4931 -> [w4941] mode=indexing
      tunnel: string[] ["STATE;", "SET;", "RH;", "T;", "AMB_RH;", "AMB_T;", "PUMP;", "FAN_IN;", "FAN_OUT;", "DEHUM;", "CURRENT;", "STALL;"] -> [w4940] mode=indexing
      tunnel: [w4939] -> w4930 mode=indexing
      n3765 = Match Pattern(string=w4941, regular expression=w4940) -> (after substring=w4939:string)  [unwired: 1 in, 3 out]
    }
    n3766 = Index Array(array=w4930) -> (element #1=→"STATE :":string, element #2=→"SET :":string, element #3=w4919:string, element #4=→"T :":string, element #5=w4917:string, element #6=→"AMB_T :":string, element #7=→"PUMP :":string, element #8=→"FAN_IN :":string, element #9=→"FAN_OUT :":string, element #10=→"DEHUM :":string, element #11=→"CURRENT :":string, element #12=→"STALL :":string)  [unwired: 12 in]
    "RH :" <- w4919
    "AMB_RH :" <- w4917
    n3767 = Fract/Exp String To Number(string=w4919) -> (number=w4912:dbl)  [unwired: 3 in, 1 out]
    n3768 = Fract/Exp String To Number(string=w4917) -> (number=w4916:dbl)  [unwired: 3 in, 1 out]
    n3769 = local write "Ambient Humidity :"(w4916) -> ()
    n3770 = Equal?(x=w4912, y=0.0) -> (x = y?=w4914:bool)
    n3771 = case shown="True" w4914 {
      tunnel: [w4937 w4938] -> w4913
      tunnel: w4912 -> [w4937 _]
      frame False {
        (unwired) 0.0
        "Humidity temp" <- w4937
      }
      frame True {
        n3772 = local read "Humidity temp"() -> (w4938:dbl)
      }
    }
    "RH Numeric:" <- w4913
    n3773 = local read "Quit"() -> (w4936:bool)
  }
  n3774 = disable-structure shown="Disabled" {
    frame Disabled {
      n3775 = while {
        tunnel: [w5175] -> _
        i -> [w5175]
        stop <- w5172 stop-if-true
        n3776 = local read "powstat"() -> (w5173:bool)
        n3777 = case shown="True" w5173 {
          frame False {
          }
          frame True {
            n3778 = local read "RUN"() -> (w5176:bool)
            n3779 = case shown="True" w5176 {
              frame False {
                w5206 = 65.0 ("y")
                n3780 = local read "Set Hz"() -> (w5234:dbl)
                n3781 = local read "NORMAL LOAD"() -> (w5235:dbl)
                n3782 = Multiply(x=w5234, y=60.0) -> (x*y=w5241:dbl)
                n3783 = Multiply(x=1.2 ("y"), y=0.949) -> (x*y=w5210:dbl)
                n3784 = Multiply(x=1.2 ("y"), y=0.8166) -> (x*y=w5214:dbl)
                n3785 = Multiply(x=1.2 ("y"), y=0.851) -> (x*y=w5209:dbl)
                n3786 = local read "FF 2"() -> (w5233:dbl)
                n3787 = Absolute Value(x=w5241) -> (abs(x)=w5239:dbl)
                n3788 = case shown="13.." w5233 {
                  tunnel: [1 2 3] -> w5231
                  frame 0..10, Default {
                    # "Normal"
                  }
                  frame 11, 12 {
                  }
                  frame 13.. {
                  }
                }
                "FF STATE" <- w5231
                n3789 = local read "TEMP"() -> (w5194:dbl)
                n3790 = local read item#-1() -> (w5208)
                n3791 = Less?(x=w5208, y=w5214) -> (x < y?=w5211:bool)
                n3792 = In Range and Coerce(upper limit=w5210, x=w5208, lower limit=w5209) -> (In Range?=w5212:bool)  [unwired: 1 out]
                n3793 = case shown="3601.." w5239 {
                  tunnel: [1 2 3] -> w5237
                  frame 0..3000, Default {
                    # "Normal"
                  }
                  frame 3001..3600 {
                  }
                  frame 3601.. {
                  }
                }
                n3794 = case shown="11.." w5235 {
                  tunnel: [1 3] -> w5236
                  frame 1..10, Default {
                  }
                  frame 11.. {
                  }
                }
                "NL STATE" <- w5236
                n3795 = Multiply(x=1.2 ("y"), y=0.95) -> (x*y=w5224:dbl)
                n3796 = Multiply(x=w5206, y=0.954) -> (x*y=w5198:dbl)
                n3797 = Or(x=w5211, y=w5212) -> (x .or. y?=w5213:bool)
                n3798 = Greater Or Equal?(x=w5208, y=w5224) -> (x >= y?=w5221:bool)
                n3799 = Multiply(x=w5206, y=0.99) -> (x*y=w5195:dbl)
                n3800 = Greater Or Equal?(x=w5194, y=w5195) -> (x >= y?=w5200:bool)
                n3801 = Greater Or Equal?(x=w5194, y=w5198) -> (x >= y?=w5197:bool)
                n3802 = case shown="0, 1, Default" w5208 {
                  tunnel: [1 3] -> w5225
                  frame 0, 1, Default {
                  }
                  frame 2.. {
                  }
                }
                n3803 = case shown="True" w5221 {
                  tunnel: [1 3] -> w5226
                  frame False {
                  }
                  frame True {
                  }
                }
                n3804 = case shown="True" w5213 {
                  tunnel: [1 2] -> w5227
                  frame False {
                  }
                  frame True {
                  }
                }
                n3805 = case shown="..0" w5194 {
                  tunnel: [2 3 3 1] -> w5201
                  frame 61, 62 {
                  }
                  frame 63.. {
                  }
                  frame ..0 {
                  }
                  frame 10..60, Default {
                  }
                }
                n3806 = case shown="True" w5200 {
                  tunnel: [1 3] -> w5202
                  frame False {
                  }
                  frame True {
                  }
                }
                n3807 = Number To Decimal String(number=w5237) -> (decimal integer string=w5238:string)  [unwired: 1 in]
                n3808 = case shown="True" w5197 {
                  tunnel: [1 2] -> w5203
                  frame False {
                  }
                  frame True {
                  }
                }
                n3809 = Number To Decimal String(number=1) -> (decimal integer string=→"Air temp":string)  [unwired: 1 in]
                n3810 = Number To Decimal String(number=w5231) -> (decimal integer string=→"ff_st":string)  [unwired: 1 in]
                n3811 = local write "sp_st"(w5238) -> ()
                n3812 = Number To Decimal String(number=w5236) -> (decimal integer string=→"nl_st":string)  [unwired: 1 in]
                n3813 = Build Array(w5201, w5202, w5203) -> (w5204:i32[])
                n3814 = Build Array(w5225, w5226, w5227) -> (w5228:i32[])
                n3815 = Array Max & Min(array=w5204) -> (max value=w5205:i32)  [unwired: 3 out]
                n3816 = Array Max & Min(array=w5228) -> (max value=w5229:i32)  [unwired: 3 out]
                n3817 = Number To Decimal String(number=w5205) -> (decimal integer string=w5193:string)  [unwired: 1 in]
                n3818 = Number To Decimal String(number=w5229) -> (decimal integer string=→"Stroke Ln 2":string)  [unwired: 1 in]
                n3819 = local write "temp_st"(w5193) -> ()
              }
              frame True {
                w5291 = 65.0 ("y")
                # "Healthy -1\nWarning -2\nError -3"
                n3820 = local read "TEMP"() -> (w5302:dbl)
                n3821 = local read "NORMAL LOAD"() -> (w5306:dbl)
                n3822 = local read "Set Hz"() -> (w5304:dbl)
                n3823 = Multiply(x=1.2 ("y"), y=0.949) -> (x*y=w5286:dbl)
                n3824 = Multiply(x=1.2 ("y"), y=0.8166) -> (x*y=w5282:dbl)
                n3825 = Multiply(x=1.2 ("y"), y=0.851) -> (x*y=w5287:dbl)
                n3826 = Multiply(x=w5291, y=0.954) -> (x*y=w5298:dbl)
                n3827 = Multiply(x=w5291, y=0.99) -> (x*y=w5301:dbl)
                n3828 = Greater Or Equal?(x=w5302, y=w5301) -> (x >= y?=w5296:bool)
                n3829 = Multiply(x=w5304, y=60.0) -> (x*y=w5310:dbl)
                n3830 = Greater Or Equal?(x=w5302, y=w5298) -> (x >= y?=w5299:bool)
                n3831 = local read "FF 2"() -> (w5305:dbl)
                n3832 = local read item#-1() -> (w5288)
                n3833 = Less?(x=w5288, y=w5282) -> (x < y?=w5285:bool)
                n3834 = In Range and Coerce(upper limit=w5286, x=w5288, lower limit=w5287) -> (In Range?=w5284:bool)  [unwired: 1 out]
                n3835 = Absolute Value(x=w5310) -> (abs(x)=w5308:dbl)
                n3836 = case shown="63.." w5302 {
                  tunnel: [2 3 3 1] -> w5295
                  frame 61, 62 {
                  }
                  frame 63.. {
                  }
                  frame ..0 {
                  }
                  frame 10..60, Default {
                  }
                }
                n3837 = case shown="True" w5296 {
                  tunnel: [1 3] -> w5294
                  frame False {
                  }
                  frame True {
                  }
                }
                n3838 = case shown="True" w5299 {
                  tunnel: [1 2] -> w5293
                  frame False {
                  }
                  frame True {
                  }
                }
                n3839 = Multiply(x=1.2 ("y"), y=0.95) -> (x*y=w5272:dbl)
                n3840 = case shown="1..10, Default" w5306 {
                  tunnel: [1 3] -> w5313
                  frame 1..10, Default {
                  }
                  frame 11.. {
                  }
                }
                n3841 = case shown="0..10, Default" w5305 {
                  tunnel: [1 2 3] -> w5312
                  frame 0..10, Default {
                  }
                  frame 11, 12 {
                  }
                  frame 13.. {
                  }
                }
                n3842 = case shown="3601.." w5308 {
                  tunnel: [1 2 3] -> w5307
                  frame 0..3000, Default {
                    # "Normal"
                  }
                  frame 3001..3600 {
                  }
                  frame 3601.. {
                  }
                }
                n3843 = Or(x=w5285, y=w5284) -> (x .or. y?=w5283:bool)
                n3844 = Greater Or Equal?(x=w5288, y=w5272) -> (x >= y?=w5275:bool)
                n3845 = case shown="0, 1, Default" w5288 {
                  tunnel: [1 3] -> w5271
                  frame 0, 1, Default {
                  }
                  frame 2.. {
                  }
                }
                n3846 = case shown="True" w5275 {
                  tunnel: [1 3] -> w5270
                  frame False {
                  }
                  frame True {
                  }
                }
                n3847 = case shown="True" w5283 {
                  tunnel: [1 2] -> w5269
                  frame False {
                  }
                  frame True {
                  }
                }
                n3848 = Build Array(w5295, w5294, w5293) -> (w5292:i32[])
                n3849 = Number To Decimal String(number=w5307) -> (decimal integer string=→"sp_st":string)  [unwired: 1 in]
                n3850 = Array Max & Min(array=w5292) -> (max value=w5289:i32)  [unwired: 3 out]
                "TEMP STATE" <- w5289
                n3851 = Number To Decimal String(number=w5313) -> (decimal integer string=w5316:string)  [unwired: 1 in]
                n3852 = Number To Decimal String(number=w5312) -> (decimal integer string=w5314:string)  [unwired: 1 in]
                n3853 = Number To Decimal String(number=w5289) -> (decimal integer string=→"temp_st":string)  [unwired: 1 in]
                n3854 = Build Array(w5271, w5270, w5269) -> (w5268:i32[])
                n3855 = local write "nl_st"(w5316) -> ()
                n3856 = local write "ff_st"(w5314) -> ()
                n3857 = Number To Decimal String(number=1) -> (decimal integer string=w5311:string)  [unwired: 1 in]
                n3858 = Array Max & Min(array=w5268) -> (max value=w5267:i32)  [unwired: 3 out]
                n3859 = local write "Air temp"(w5311) -> ()
                n3860 = Number To Decimal String(number=w5267) -> (decimal integer string=w5266:string)  [unwired: 1 in]
                n3861 = local write "Stroke Ln 2"(w5266) -> ()
              }
            }
            n3862 = local read "Stroke Ln 2"() -> (w5178:string)
            n3863 = local read "nl_st"() -> (w5184:string)
            n3864 = local read "ff_st"() -> (w5181:string)
            n3865 = local read "sp_st"() -> (w5182:string)
            n3866 = local read "temp_st"() -> (w5183:string)
            n3867 = local read "Air temp"() -> (w5177:string)
            n3868 = Replace Array Subset(array="in", new element #1=w5184, index #1=1 ("index"), new element #2=w5181, index #2=2 ("index"), new element #3=w5183, index #3=3 ("index"), new element #4=w5182, index #4=4 ("index"), new element #5=w5178, index #5=5 ("index"), new element #6=w5177, index #6=6 ("index"), new element #7="Sensor State" ("new element/subarray"), index #7=0 ("index")) -> (→"out":string[])
          }
        }
        n3869 = Wait (ms)(milliseconds to wait=u32 10) -> ()  [unwired: 1 out]
        n3870 = local read "Quit"() -> (w5172:bool)
      }
      n3871 = while {
        stop <- w5147 stop-if-true
        n3872 = local read "run replace"() -> (w5149:bool)
        n3873 = Wait (ms)(milliseconds to wait=u32 100) -> ()  [unwired: 1 out]
        n3874 = Equal?(x="FLAG 2", y=0.0) -> (x = y?=w5150:bool)
        n3875 = case shown="True" w5150 {
          frame False {
          }
          frame True {
            n3876 = local write "FLAG 2"(100.0 ("FLAG 2")) -> ()
            n3877 = call <vilib>:"Read Characters From File.vi"("file path (dialog if empty)"=path "C:/LAB-IQ-NXT/WO 2449 TT.sig", "convert eol? (no:F)"=FALSE ("append to file? (new file:F)")) -> ("character string"=w5153:string)  [unwired: 4 in, 3 out]
            n3878 = call <vilib>:"Read Characters From File.vi"("file path (dialog if empty)"=path "C:/LAB-IQ-NXT/WO 2449 TRH.sig", "convert eol? (no:F)"=FALSE ("append to file? (new file:F)")) -> ("character string"=w5154:string)  [unwired: 4 in, 3 out]
            n3879 = Decimal String To Number(string=w5153) -> (number=w5155:i32)  [unwired: 2 in, 1 out]
            n3880 = local write "Total No. of Tests"(w5155) -> ()
            n3881 = Decimal String To Number(string=w5154) -> (number=w5158:i32)  [unwired: 2 in, 1 out]
            n3882 = local write "SEN.RUN HRS"(w5158) -> ()
          }
        }
        n3883 = case shown="True" w5149 {
          frame False {
          }
          frame True {
            n3884 = Equal?(x="FLAG 4", y=0.0) -> (x = y?=w5162:bool)
            n3885 = case shown="False" w5162 {
              frame False {
                n3886 = Get Date/Time In Seconds() -> (seconds since 1Jan1904=w5168:timestamp)
                n3887 = local read "START 3"() -> (w5166:dbl)
                n3888 = To Double Precision Float(number=w5168) -> (double precision float=w5167:dbl)
                n3889 = Subtract(x=w5167, y=w5166) -> (x-y=→"SENSOR TIME":dbl)
              }
              frame True {
                n3890 = Get Date/Time In Seconds() -> (seconds since 1Jan1904=w5170:timestamp)
                n3891 = local write "FLAG 4"(100.0 ("FLAG")) -> ()
                n3892 = To Double Precision Float(number=w5170) -> (double precision float=→"START 3":dbl)
              }
            }
          }
        }
        n3893 = local read "Quit"() -> (w5147:bool)
      }
      n3894 = while {
        shift-right: [w4947] -> _
        shift-left: _ -> [w4948]
        tunnel: [w4943] -> _
        i -> [w4943]
        stop <- w4942 stop-if-true
        n3895 = Wait (ms)(milliseconds to wait=u32 50 ("Refresh Rate (ms)")) -> ()  [unwired: 1 out]
        n3896 = local read "Json End Flg"() -> (w4944:bool)
        n3897 = Not(x="Upld AR 2") -> ()  [unwired: 1 out]
        n3898 = local read "Upld AR 2"() -> (w4945:bool)
        n3899 = call "Elapsed Time9"("Time Target (s)"="Sen.Upload Rate (s)", "Reset"=FALSE, "Auto Reset"=TRUE) -> ("Time has Elapsed"=w4954:bool)  [unwired: 9 in, 7 out]
        n3900 = Or(x=w4954, y=w4944) -> (x .or. y?=w4950:bool)
        n3901 = case shown="True" w4950 {
          frame False {
          }
          frame True {
            w5046 = "\"SensorName\":\"" ("string")
            w5016 = " \"},{"
            w5041 = "\",\"SensorState\":\""
            w5043 = "\",\"SensorModelNumber\":\"" ("string")
            w5042 = "\",\"SensorRuntimeHours\":\"" ("string")
            n3902 = local read "model num"() -> (w5040:string[])
            n3903 = local read "Sensor name"() -> (w5059:string[])
            n3904 = local read "run"() -> (w5030:string[])
            n3905 = local read "SENSOR TIME"() -> (w4986:dbl)
            n3906 = local read "out"() -> (w4979:string[])
            n3907 = local read "Total No. of Tests"() -> (w4984:dbl)
            n3908 = Select(t=60.0, s="Run test 3", f=3600.0) -> (s? t:f=w4994:dbl)
            n3909 = Index Array(array=w5040, index #1=1 ("index")) -> (element #1=w5039:string, element #2=w5038:string, element #3=w5037:string, element #4=w5036:string, element #5=w5035:string, element #6=w5034:string)  [unwired: 5 in]
